vi "AIT 664 Parameter Page.vi"(8 "error in (no error)":errorcluster, 11 "Node Ptr":T3 format="%.0x") -> (0 "error out":errorcluster)   [LabVIEW 2013, in "AIT 664 Custom Device.lvlib"]
uses:
  AIT 664 Custom Device.lvlib
  <vilib>/NI Veristand/Custom Device API/Custom Device Item Ref.ctl
  Controls and Global/Start Bit.ctl
  Controls and Global/Number of Bits.ctl
  Controls/664 -Param.ctl
  Controls and Global/Global.vi
  <vilib>/NI Veristand/Custom Device API/Get Item Property (U32 Array).vi
  <vilib>/NI Veristand/Custom Device API/Get Item Property (Boolean).vi
  <vilib>/NI Veristand/Custom Device API/Get Item Property (U16).vi
  <vilib>/NI Veristand/Custom Device API/Get Item Property (Double).vi
  <vilib>/NI Veristand/Custom Device API/Get Item Property (I32).vi
  <vilib>/NI Veristand/Custom Device API/Set Item Property (U16).vi
  <vilib>/NI Veristand/Custom Device API/Set Item Property (I32).vi
  <vilib>/NI Veristand/Custom Device API/Set Item Property (Boolean).vi
  <vilib>/NI Veristand/Custom Device API/Set Item Property (Double).vi
  <vilib>/NI Veristand/Custom Device API/Custom Device API.lvlib
panel:
  in  "First Byte":u16
  out "TriggerDValChange":bool
  in  "Scale Offset":dbl format="%#_6f"
  in  "Scale Factor":dbl format="%#_6f"
  in  "Signed?":bool
  out "Default Value":dbl
  in  "Number of Bits":T1=1 min=1 max=32
  in  "Start Bit":T2=1
  in  "Header":cluster{"Section Name":string}={"Section Name"="AIT 664  Parameter"}
  in  "Description":string
  in  "Name":string
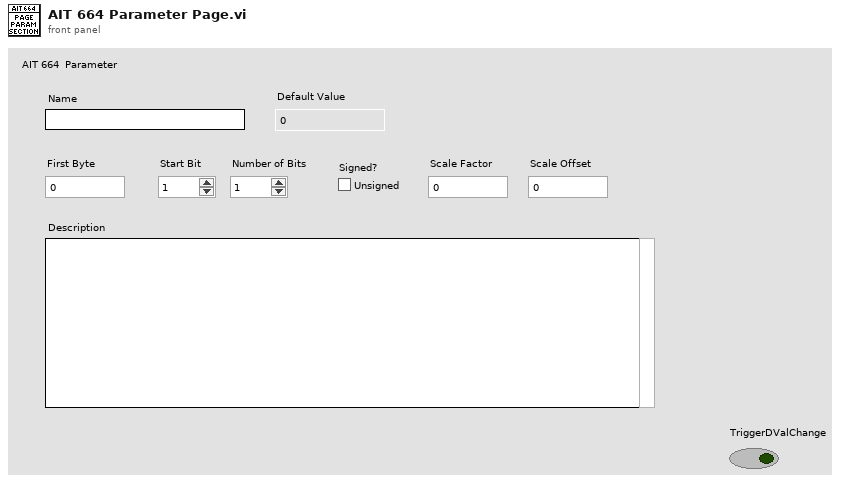
[diagram p1: front panel]
types:
  T1 = typedef "AIT 664 Custom Device.lvlib/Number of Bits.ctl" = i32
  T2 = typedef "AIT 664 Custom Device.lvlib/Start Bit.ctl" = i32
  T3 = typedef "Custom Device API.lvlib/Custom Device Item Ref.ctl" = u64
  T4 = typedef "Custom Device API.lvlib/Custom Device Item Info.ctl" = cluster{"Name":string, "Is Channel":bool, "GUID":string, "Is Waveform":bool}
  T5 = typedef "Custom Device API.lvlib/Custom Device Channel.ctl" = cluster{"Type":T6, "Units":string, "Default Value":dbl, "Faultable":bool, "Scalable":bool}
  T6 = typedef "Custom Device API.lvlib/Custom Device Channel Type.ctl" = enum16{"Input", "Output"}
  T7 = typedef "AIT 664 Custom Device.lvlib/664 -Param.ctl" = cluster{"name":string, "firstByte":i32, "startBit":i32, "numberBits":i32, "scaleFactor":dbl, "scaleOffset":dbl, "signed":bool}
  T8 = typedef "Custom Device API.lvlib/Custom Device Commands.ctl" = enum16{"Default", "Item renamed", "Shutdown", "Dynamic button pressed"}
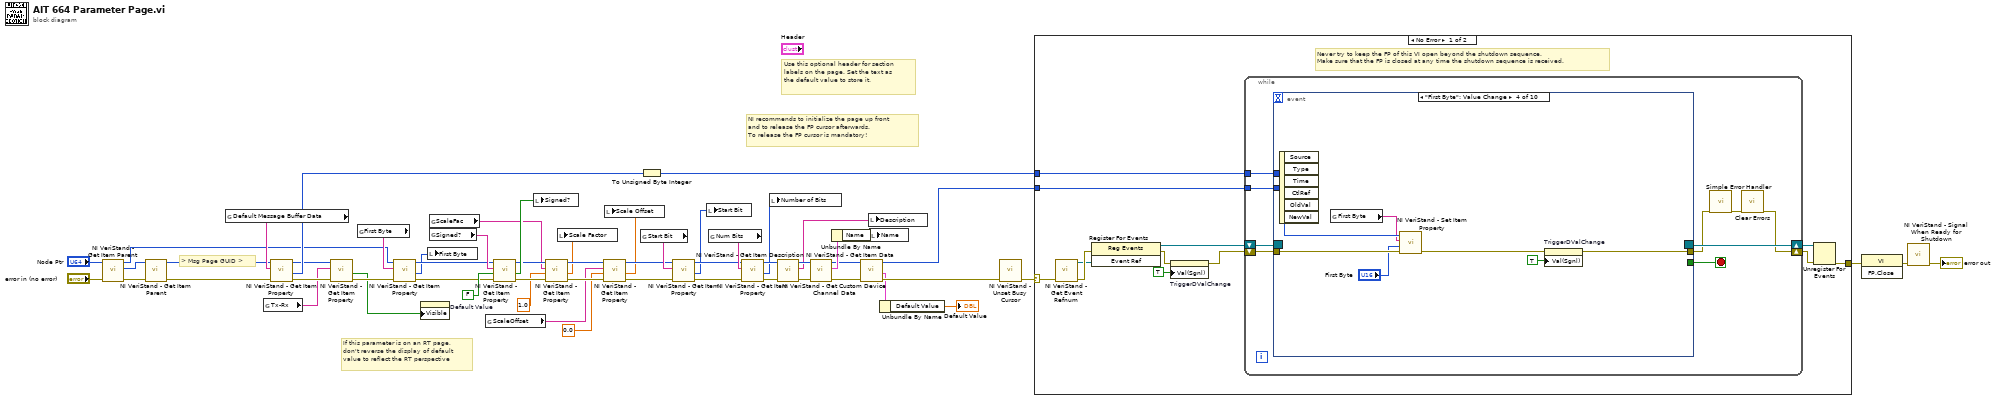
[diagram p0: block diagram]
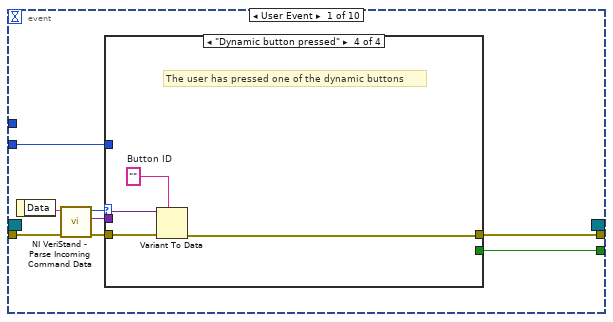
[diagram p2: hidden frame]
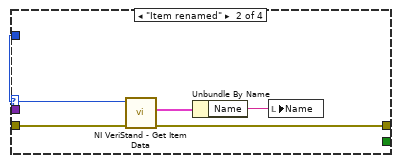
[diagram p4: hidden frame]
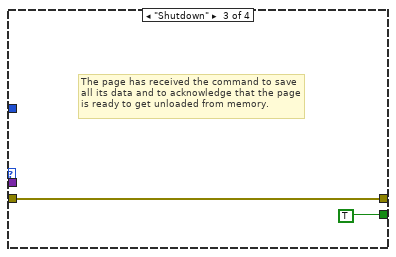
[diagram p5: hidden frame]
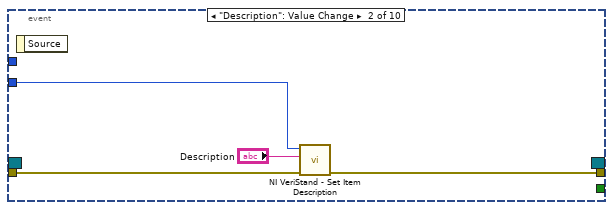
[diagram p6: hidden frame]
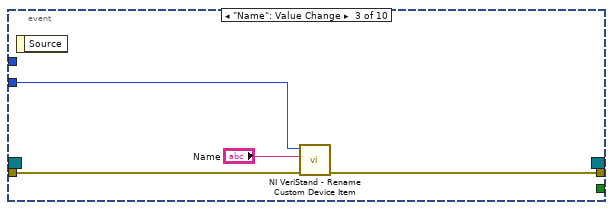
[diagram p7: hidden frame]
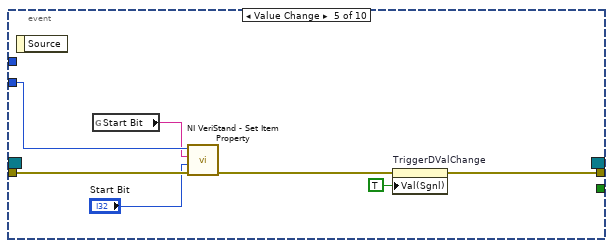
[diagram p8: hidden frame]
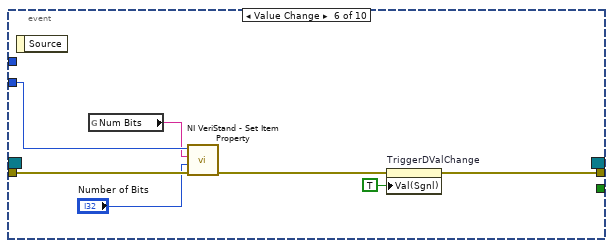
[diagram p9: hidden frame]
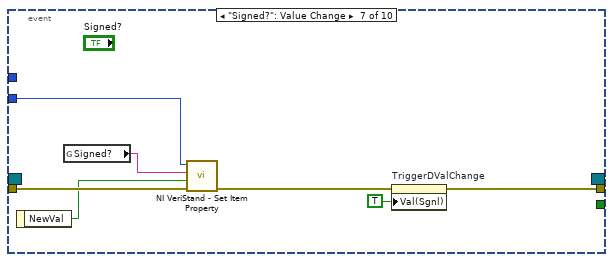
[diagram p10: hidden frame]
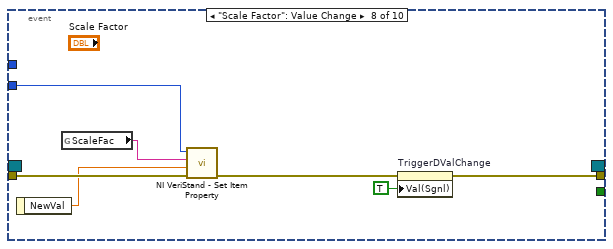
[diagram p11: hidden frame]
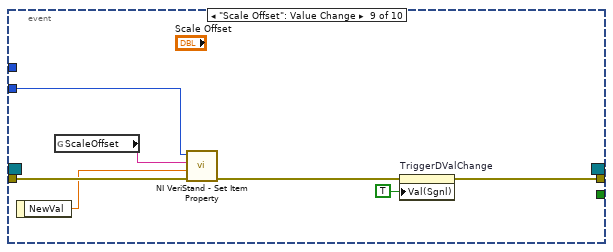
[diagram p12: hidden frame]
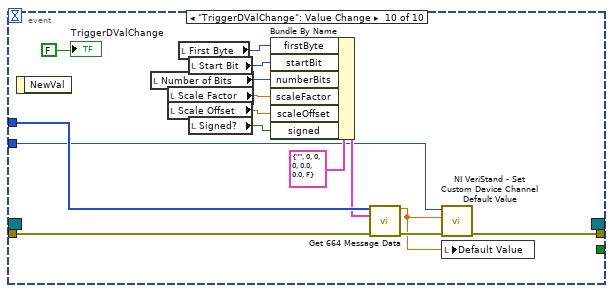
[diagram p13: hidden frame]
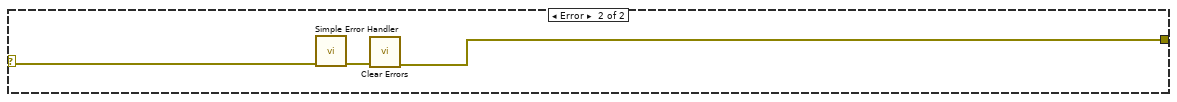
[diagram p14: hidden frame]
diagram:
  # "> Msg Page GUID >"
  # "If this parameter is on an RT page, \ndon't reverse the display of default\nvalue to reflect the RT perspective"
  # "Use this optional header for section labels on the page. Set the text as the default value to store it."
  # "NI recommends to initialize the page up front\nand to release the FP cursor afterwards.\nTo release the FP cursor is mandatory!"
  n1 = call <vilib>:"NI VeriStand - Get Item Parent.vi"("error in (no error)"="error in (no error)", "Item Ref in"="Node Ptr") -> ("error out"=w5:errorcluster, "Parent Ref"=w6:T3, "Item Ref out"=w4:T3)  [unwired: 6 in, 1 out]
  n2 = call <vilib>:"NI VeriStand - Get Item Parent.vi"("error in (no error)"=w5, "Item Ref in"=w6) -> ("error out"=w1:errorcluster, "Item Ref out"=w3:T3)  [unwired: 6 in, 2 out]
  n3 = global read "Global.vi" "Default Message Buffer Data"() -> (w34:string)
  n4 = global read "Global.vi" "Tx-Rx"() -> (w10:string)
  n5 = call-poly <vilib>:"NI VeriStand - Get Item Property.vi"("error in (no error)"=w1, "Property Name"=w34, "Item Ref in"=w3) -> ("error out"=w11:errorcluster, "Value"=w33:u32[], "Item Ref out"=w9:T3)  [unwired: 5 in, 1 out]
  n6 = call-poly <vilib>:"NI VeriStand - Get Item Property.vi"("error in (no error)"=w11, "Property Name"=w10, "Item Ref in"=w9) -> ("error out"=w8:errorcluster, "Value"=w2:bool)  [unwired: 5 in, 2 out]
  n7 = global read "Global.vi" "First Byte"() -> (w13:string)
  n8 = call-poly <vilib>:"NI VeriStand - Get Item Property.vi"("error in (no error)"=w8, "Property Name"=w13, "Item Ref in"=w4) -> ("error out"=w15:errorcluster, "Value"=w12:u16, "Item Ref out"=w14:T3)  [unwired: 5 in, 1 out]
  n9 = property on="Default Value" class="DigNum (strict)"("Visible"=w2) -> ()  [unwired: 2 in, 2 out]
  n10 = local write "First Byte"(w12) -> ()
  n11 = global read "Global.vi" "ScaleFac"() -> (w18:string)
  n12 = global read "Global.vi" "Signed?"() -> (w32:string)
  n13 = global read "Global.vi" "ScaleOffset"() -> (w22:string)
  n14 = call-poly <vilib>:"NI VeriStand - Get Item Property.vi"("error in (no error)"=w15, "Default Value"=FALSE, "Property Name"=w32, "Item Ref in"=w14) -> ("error out"=w29:errorcluster, "Value"=w30:bool, "Item Ref out"=w28:T3)  [unwired: 4 in, 1 out]
  n15 = local write "Signed?"(w30) -> ()
  n16 = call-poly <vilib>:"NI VeriStand - Get Item Property.vi"("error in (no error)"=w29, "Default Value"=1.0 ("Scale Factor"), "Property Name"=w18, "Item Ref in"=w28) -> ("error out"=w26:errorcluster, "Value"=w17:dbl, "Item Ref out"=w25:T3)  [unwired: 4 in, 1 out]
  n17 = local write "Scale Factor"(w17) -> ()
  n18 = call-poly <vilib>:"NI VeriStand - Get Item Property.vi"("error in (no error)"=w26, "Default Value"=0.0 ("Scale Factor"), "Property Name"=w22, "Item Ref in"=w25) -> ("error out"=w24:errorcluster, "Value"=w20:dbl, "Item Ref out"=w23:T3)  [unwired: 4 in, 1 out]
  n19 = local write "Scale Offset"(w20) -> ()
  n20 = To Unsigned Byte Integer(number=w33) -> (unsigned 8bit integer=w19:u8[])
  n21 = global read "Global.vi" "Start Bit"() -> (w45:string)
  n22 = call-poly <vilib>:"NI VeriStand - Get Item Property.vi"("error in (no error)"=w24, "Property Name"=w45, "Item Ref in"=w23) -> ("error out"=w43:errorcluster, "Value"=w42:i32, "Item Ref out"=w44:T3)  [unwired: 5 in, 1 out]
  n23 = local write "Start Bit"(w42) -> ()
  n24 = global read "Global.vi" "Num Bits"() -> (w48:string)
  n25 = call-poly <vilib>:"NI VeriStand - Get Item Property.vi"("error in (no error)"=w43, "Property Name"=w48, "Item Ref in"=w44) -> ("error out"=w46:errorcluster, "Value"=w41:i32, "Item Ref out"=w47:T3)  [unwired: 5 in, 1 out]
  n26 = local write "Number of Bits"(w41) -> ()
  n27 = call <vilib>:"NI VeriStand - Get Item Description.vi"("error in (no error)"=w46, "Item Ref in"=w47) -> ("error out"=w51:errorcluster, "Description"=w52:string, "Item Ref out"=w53:T3)  [unwired: 7 out]
  n28 = call <vilib>:"NI VeriStand - Get Item Data.vi"("error in (no error)"=w51, "Item Ref in"=w53) -> ("error out"=w38:errorcluster, "Item Info"=w50:T4, "Item Ref out"=w37:T3)  [unwired: 7 out]
  n29 = Unbundle By Name(w50) -> ("Name"=w49:string)
  n30 = call <vilib>:"NI VeriStand - Get Custom Device Channel Data.vi"("error in (no error)"=w38, "Channel Ref in"=w37) -> ("error out"=w36:errorcluster, "Channel"=w35:T5, "Channel Ref out"=w7:T3)  [unwired: 4 in, 3 out]
  n31 = local write "Description"(w52) -> ()
  n32 = local write "Name"(w49) -> ()
  n33 = Unbundle By Name(w35) -> ("Default Value"=→"Default Value":dbl)
  n34 = call <vilib>:"NI VeriStand - Unset Busy Cursor.vi"("error in (no error)"=w36) -> ("error out"=w54:errorcluster)  [unwired: 10 out]
  n35 = case shown="No Error" w54 {
    selector: w54 -> [w62 w166]
    tunnel: [w66 w164] -> w57
    tunnel: w7 -> [w63 _]
    tunnel: w19 -> [w61 _]
    frame No Error {
      # "Never try to keep the FP of this VI open beyond the shutdown sequence.\nMake sure that the FP is closed at any time the shutdown sequence is received."
      n36 = call <vilib>:"NI VeriStand - Get Event Refnum.vi"("error in (no error)"=w62) -> ("error out"=w69:errorcluster, "Event Ref"=w65:refnum<user-event>)  [unwired: 9 out]
      n37 = register-events(error in=w69, w65) -> (reference out=w64:refnum<event-registration>, error out=w59:errorcluster)  [unwired: 1 in]
      n38 = property on="TriggerDValChange" class="Bool (strict)"(error in=w59, "Val(Sgnl)"=TRUE ("Value (Signaling)")) -> (error out=w58:errorcluster)  [unwired: 1 in, 1 out]
      n39 = while {
        tunnel: w63 -> [w74]
        shift-right: [w71] -> w67
        shift-left: w58 -> [w77]
        shift-right: [w78] -> w68
        shift-left: w64 -> [w76]
        tunnel: w61 -> [w70]
        stop <- w75 stop-if-true
        n40 = event shown="[3] \"First Byte\": Value Change" {
          selector: w76 -> [_ _ _ _ _ _ _ _ _ _]
          dyn-events: [_ _ _ _ _ _ _ _ _ _] -> w78
          timeout: _ -> [_ _ _ _ _ _ _ _ _ _]
          tunnel: w77 -> [w86 w101 w105 w113 w120 w127 w134 w141 w148 w152]
          tunnel: [w82 _ _ _ _ _ _ _ _ _] -> w75
          tunnel: [w81 w100 w104 w109 w116 w121 w128 w135 w142 w163] -> w73
          tunnel: w74 -> [w80 w102 w106 w112 w119 w126 w133 w140 w147 w150]
          tunnel: w70 -> [_ _ _ _ _ _ _ _ _ w161]
          event User Event {
            n41 = event-data() -> ("Data"=w85:string)  [unwired: 1 out]
            n42 = call <vilib>:"NI VeriStand - Parse Incoming Command Data.vi"("error in (no error)"=w86, "Incoming data"=w85) -> ("error out"=w84:errorcluster, "Outgoing data"=w79:variant, "Action"=w83:T8)  [unwired: 7 out]
            n43 = case shown="\"Dynamic button pressed\"" w83 {
              tunnel: w84 -> [w87 w92 w93 w98]
              tunnel: [_ _ TRUE _] -> w82
              tunnel: [w87 w89 w93 w95] -> w81
              tunnel: w80 -> [_ w91 _ _]
              tunnel: w79 -> [_ _ _ w97]
              frame "Default", Default {
              }
              frame "Item renamed" {
                n44 = call <vilib>:"NI VeriStand - Get Item Data.vi"("error in (no error)"=w92, "Item Ref in"=w91) -> ("error out"=w89:errorcluster, "Item Info"=w90:T4)  [unwired: 8 out]
                n45 = Unbundle By Name(w90) -> ("Name"=w88:string)
                n46 = local write "Name"(w88) -> ()
              }
              frame "Shutdown" {
                # "The page has received the command to save all its data and to acknowledge that the page is ready to get unloaded from memory."
              }
              frame "Dynamic button pressed" {
                w96 = ""  # Button ID
                # "The user has pressed one of the dynamic buttons"
                n47 = Variant To Data(error in=w98, type=w96, Variant=w97) -> (error out=w95:errorcluster)  [unwired: 1 out]
              }
            }
          }
          event "Description": Value Change {
            n48 = event-data() -> ()  [unwired: 2 out]
            n49 = call <vilib>:"NI VeriStand - Set Item Description.vi"("error in (no error)"=w101, "Description"="Description", "Item Ref in"=w102) -> ("error out"=w100:errorcluster)  [unwired: 8 out]
          }
          event "Name": Value Change {
            n50 = event-data() -> ()  [unwired: 2 out]
            n51 = call <vilib>:"NI VeriStand - Rename Custom Device Item.vi"("error in (no error)"=w105, "New Name"="Name", "Item Ref in"=w106) -> ("error out"=w104:errorcluster)  [unwired: 6 in, 2 out]
          }
          event "First Byte": Value Change {
            n52 = event-data() -> ()  [unwired: 7 out]
            n53 = global read "Global.vi" "First Byte"() -> (w111:string)
            n54 = call-poly <vilib>:"NI VeriStand - Set Item Property.vi"("error in (no error)"=w113, "Value"="First Byte", "Property Name"=w111, "Item Ref in"=w112) -> ("error out"=w110:errorcluster)  [unwired: 5 in, 2 out]
            n55 = property on="TriggerDValChange" class="Bool (strict)"(error in=w110, "Val(Sgnl)"=TRUE ("Value (Signaling)")) -> (error out=w109:errorcluster)  [unwired: 1 in, 1 out]
          }
          event Value Change {
            n56 = event-data() -> ()  [unwired: 2 out]
            n57 = global read "Global.vi" "Start Bit"() -> (w118:string)
            n58 = call-poly <vilib>:"NI VeriStand - Set Item Property.vi"("error in (no error)"=w120, "Value"="Start Bit", "Property Name"=w118, "Item Ref in"=w119) -> ("error out"=w117:errorcluster)  [unwired: 5 in, 2 out]
            n59 = property on="TriggerDValChange" class="Bool (strict)"(error in=w117, "Val(Sgnl)"=TRUE ("Value (Signaling)")) -> (error out=w116:errorcluster)  [unwired: 1 in, 1 out]
          }
          event Value Change {
            n60 = event-data() -> ()  [unwired: 2 out]
            n61 = global read "Global.vi" "Num Bits"() -> (w125:string)
            n62 = call-poly <vilib>:"NI VeriStand - Set Item Property.vi"("error in (no error)"=w127, "Value"="Number of Bits", "Property Name"=w125, "Item Ref in"=w126) -> ("error out"=w122:errorcluster)  [unwired: 5 in, 2 out]
            n63 = property on="TriggerDValChange" class="Bool (strict)"(error in=w122, "Val(Sgnl)"=TRUE ("Value (Signaling)")) -> (error out=w121:errorcluster)  [unwired: 1 in, 1 out]
          }
          event "Signed?": Value Change {
            n64 = event-data() -> ("NewVal"=w131:bool)  [unwired: 1 out]
            n65 = global read "Global.vi" "Signed?"() -> (w132:string)
            n66 = call-poly <vilib>:"NI VeriStand - Set Item Property.vi"("error in (no error)"=w134, "Value"=w131, "Property Name"=w132, "Item Ref in"=w133) -> ("error out"=w129:errorcluster)  [unwired: 5 in, 2 out]
            n67 = property on="TriggerDValChange" class="Bool (strict)"(error in=w129, "Val(Sgnl)"=TRUE ("Value (Signaling)")) -> (error out=w128:errorcluster)  [unwired: 1 in, 1 out]
          }
          event "Scale Factor": Value Change {
            n68 = event-data() -> ("NewVal"=w138:dbl)  [unwired: 1 out]
            n69 = global read "Global.vi" "ScaleFac"() -> (w139:string)
            n70 = call-poly <vilib>:"NI VeriStand - Set Item Property.vi"("error in (no error)"=w141, "Value"=w138, "Property Name"=w139, "Item Ref in"=w140) -> ("error out"=w136:errorcluster)  [unwired: 5 in, 2 out]
            n71 = property on="TriggerDValChange" class="Bool (strict)"(error in=w136, "Val(Sgnl)"=TRUE ("Value (Signaling)")) -> (error out=w135:errorcluster)  [unwired: 1 in, 1 out]
          }
          event "Scale Offset": Value Change {
            n72 = event-data() -> ("NewVal"=w145:dbl)  [unwired: 1 out]
            n73 = global read "Global.vi" "ScaleOffset"() -> (w146:string)
            n74 = call-poly <vilib>:"NI VeriStand - Set Item Property.vi"("error in (no error)"=w148, "Value"=w145, "Property Name"=w146, "Item Ref in"=w147) -> ("error out"=w143:errorcluster)  [unwired: 5 in, 2 out]
            n75 = property on="TriggerDValChange" class="Bool (strict)"(error in=w143, "Val(Sgnl)"=TRUE ("Value (Signaling)")) -> (error out=w142:errorcluster)  [unwired: 1 in, 1 out]
          }
          event "TriggerDValChange": Value Change {
            n76 = event-data() -> ()  [unwired: 2 out]
            n77 = local read "Number of Bits"() -> (w158:T1)
            n78 = local read "Scale Factor"() -> (w157:dbl)
            n79 = local read "Scale Offset"() -> (w156:dbl)
            n80 = local read "First Byte"() -> (w154:u16)
            n81 = local read "Start Bit"() -> (w159:T2)
            n82 = local read "Signed?"() -> (w153:bool)
            n83 = Bundle By Name(cluster=T7 {"name"="", "firstByte"=0, "startBit"=0, "numberBits"=0, "scaleFactor"=0.0, "scaleOffset"=0.0, "signed"=FALSE} ("1553 Parameter"), "firstByte"=w154, "startBit"=w159, "numberBits"=w158, "scaleFactor"=w157, "scaleOffset"=w156, "signed"=w153) -> (w155:T7)
            n84 = call "Get 664 Message Data.vi"("MSG DATA"=w161, "664 Parameter"=w155, "error in (no error)"=w152) -> ("Value"=w149:dbl, "error out"=w151:errorcluster)  [unwired: 11 in]
            n85 = call <vilib>:"NI VeriStand - Set Custom Device Channel Default Value.vi"("error in (no error)"=w151, "Default Value"=w149, "Channel Ref in"=w150) -> ("error out"=w163:errorcluster)  [unwired: 7 in, 1 out]
            n86 = local write "Default Value"(w149) -> ()
            "TriggerDValChange" <- FALSE
          }
        }
        n87 = call <vilib>:"Simple Error Handler.vi"("error in (no error)"=w73) -> ("error out"=w72:errorcluster)  [unwired: 1 in, 7 out]
        n88 = call <vilib>:"Clear Errors.vi"("error in (no error)"=w72) -> ("error out"=w71:errorcluster)  [unwired: 6 out]
      }
      n89 = Unregister For Events(event registration refnum=w68, error in=w67) -> (error out=w66:errorcluster)
    }
    frame Error {
      n90 = call <vilib>:"Simple Error Handler.vi"("error in (no error)"=w166) -> ("error out"=w165:errorcluster)  [unwired: 1 in, 7 out]
      n91 = call <vilib>:"Clear Errors.vi"("error in (no error)"=w165) -> ("error out"=w164:errorcluster)  [unwired: 6 out]
    }
  }
  n92 = invoke class="VI" method="FP.Close"(error in=w57) -> (error out=w56:errorcluster)  [unwired: 2 in, 2 out]
  n93 = call <vilib>:"NI VeriStand - Signal When Ready for Shutdown.vi"("error in (no error)"=w56) -> ("error out"=→"error out":errorcluster)  [unwired: 10 out]
